vi "TemplateGUI_MainGUIActive.vi"(8 "ErrorIn":errorcluster, 11 "ReferenceIn":refnum<class "TemplateGUI.lvclass">) -> (0 "ErrorOut":errorcluster, 3 "ReferenceIn":refnum<class "TemplateGUI.lvclass">)   [LabVIEW 2021, in "TemplateGUIOpenGDSActiveObject.lvlib" / "TemplateGUI.lvclass"]
uses:
  TemplateGUI.lvclass
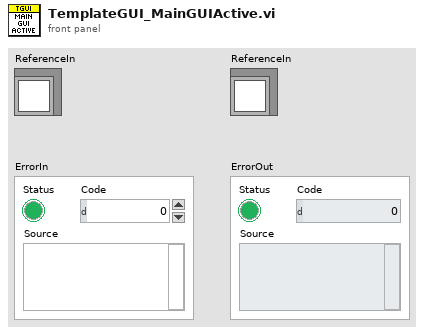
[diagram p1: front panel]
types:
  T1 = typedef "TemplateGUI.lvlib/TemplateGUI.lvclass/ObjectAttributes.ctl" = cluster{"Interfaces":cluster{"Dummys":refnum<class>}, "Locals":cluster{"MainGUIActive":refnum<queue>}, "Persistent":cluster{"Dummy":bool}}
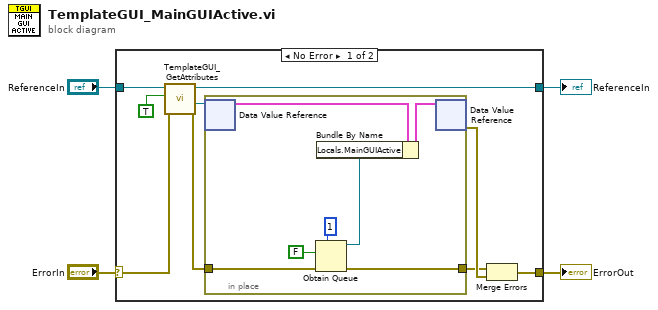
[diagram p0: block diagram]
diagram:
  n1 = case shown="No Error" "ErrorIn" {
    selector: "ErrorIn" -> [w13 w22]
    tunnel: [w11 w22] -> w3
    tunnel: [w7 w21] -> w1
    tunnel: "ReferenceIn" -> [w8 w21]
    frame No Error {
      n2 = call "TemplateGUI_GetAttributes.vi"("ErrorIn"=w13, "OnlyGetDvrReference(False)"=TRUE, "ReferenceIn"=w8) -> ("ErrorOut"=w10:errorcluster, "DataRef"=w5:refnum<data-value>, "ReferenceOut"=w7:refnum<class "TemplateGUI.lvclass">)  [unwired: 5 in, 1 out]
      n3 = in-place {
        in-place-border: w10 -> [w20]
        in-place-border: [w19] -> w9
        n4 = in-place-dvr #1(w5) -> (w17:T1)  [unwired: 1 out]
        n5 = Obtain Queue(max queue size (-1, unlimited)=1, element data type=FALSE, error in (no error)=w20) -> (queue out=w14:refnum<queue>, error out=w19:errorcluster)  [unwired: 2 in, 1 out]
        n6 = Bundle By Name(cluster=w17, "Locals.MainGUIActive"=w14) -> (w18:T1)
        n7 = in-place-dvr #1(w18) -> (w12:errorcluster)  [unwired: 1 out]
      }
      n8 = Merge Errors(w9, w12) -> (w11:errorcluster)
    }
    frame Error {
    }
  }
  "ErrorOut" <- w3
  "ReferenceIn" <- w1
